vi "Filter List - Workspace.vi"(6 "Filter results:":enum32{"Radio Selection 2", "Radio Selection 1"}(radio), 7 "error in (no error)":errorcluster, 8 "CaseSens":bool, 9 "Filter String":string, 10 "names list in":string[](array[string])) -> (0 "error out":errorcluster, 3 "names list out":string[](array[string]))   [LabVIEW 2011]
uses:
  <userlib>/_OpenG.lib/array/array.llb/Filter 1D Array with Scalar (String)__ogtk.vi
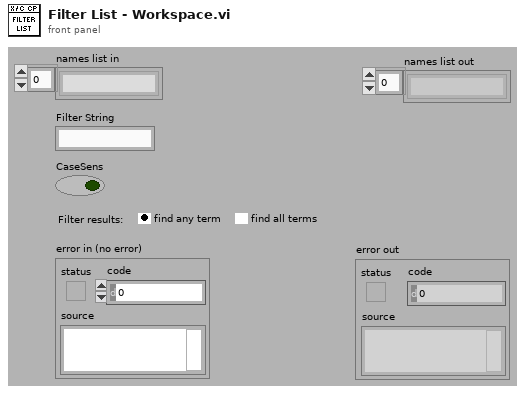
[diagram p1: front panel]
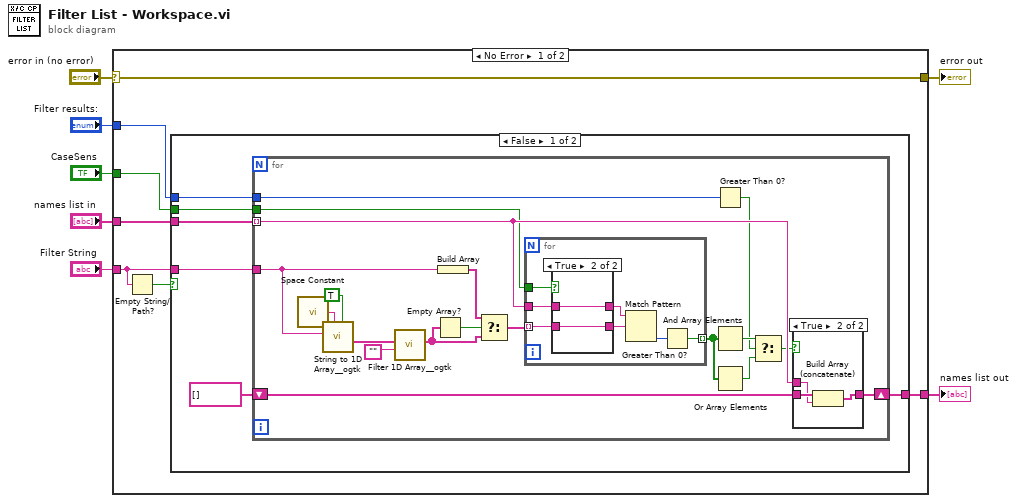
[diagram p0: block diagram]
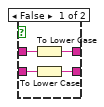
[diagram p2: hidden frame]
diagram:
  n1 = case shown="No Error" "error in (no error)" {
    selector: "error in (no error)" -> [w8 w58]
    tunnel: "CaseSens" -> [w14 _]
    tunnel: "Filter String" -> [w13 _]
    tunnel: [w11 _] -> w5
    tunnel: "names list in" -> [w10 _]
    tunnel: "Filter results:" -> [w9 _]
    tunnel: [w8 w58] -> w1
    frame No Error {
      n2 = Empty String/Path?(string/path=w13) -> (empty?=w12:bool)
      n3 = case shown="False" w12 {
        tunnel: w10 -> [w20 w57]
        tunnel: [w18 w57] -> w11
        tunnel: w13 -> [w17 _]
        tunnel: w14 -> [w16 _]
        tunnel: w9 -> [w15 _]
        frame False {
          n4 = for {
            tunnel: w20 -> [w37] mode=indexing
            tunnel: w17 -> [w25]
            shift-right: [w38] -> w18
            shift-left: string[] [] ("names list out") -> [w39]
            tunnel: w16 -> [w36]
            tunnel: w15 -> [w21]
            n5 = call <vilib>:"Space Constant.vi"() -> ("String"=w35:string)
            n6 = call <userlib>:"String to 1D Array__ogtk.vi"("ignore duplicate delimiters? (F=No)"=TRUE, "delimiter (Tab)"=w35, "string"=w25) -> ("Array of Strings"=w29:string[])  [unwired: 8 in]
            n7 = call-poly <userlib>:"Filter 1D Array__ogtk.vi"("items to filter"="", "array"=w29) -> ("filtered array"=w26:string[])  [unwired: 4 in, 1 out]
            n8 = Empty Array?(array=w26) -> (empty?=w27:bool)
            n9 = Build Array(w25) -> (w24:string[])
            n10 = Select(t=w24, s=w27, f=w26) -> (s? t:f=w23:string[])
            n11 = for {
              tunnel: w23 -> [w45] mode=indexing
              tunnel: [w42] -> w33 mode=indexing
              tunnel: w37 -> [w41]
              tunnel: w36 -> [w40]
              n12 = case shown="True" w40 {
                tunnel: [w50 w51] -> w44
                tunnel: w41 -> [w49 w51]
                tunnel: w45 -> [w48 w52]
                tunnel: [w47 w52] -> w43
                frame False {
                  n13 = To Lower Case(string=w49) -> (all lower case string=w50:string)
                  n14 = To Lower Case(string=w48) -> (all lower case string=w47:string)
                }
                frame True {
                }
              }
              n15 = Match Pattern(string=w44, regular expression=w43) -> (offset past match=w46:i32)  [unwired: 1 in, 3 out]
              n16 = Greater Than 0?(x=w46) -> (x > 0?=w42:bool)
            }
            n17 = Greater Than 0?(x=w21) -> (x > 0?=w22:bool)
            n18 = And Array Elements(Boolean array=w33) -> (logical AND=w31:bool)
            n19 = Or Array Elements(Boolean array=w33) -> (logical OR=w32:bool)
            n20 = Select(t=w31, s=w22, f=w32) -> (s? t:f=w30:bool)
            n21 = case shown="True" w30 {
              tunnel: w39 -> [w53 w56]
              tunnel: [w53 w55] -> w38
              tunnel: w37 -> [_ w54]
              frame False {
              }
              frame True {
                n22 = Build Array (concatenate)(w56, w54) -> (w55:string[])
              }
            }
          }
        }
        frame True {
        }
      }
    }
    frame Error {
    }
  }
  "names list out" <- w5
  "error out" <- w1
